vi "load_calib_file.vi"(0 "file_1":path, 1 "file_2":path, 2 "transpose? (F)":bool, 3 "delimiter (;)":string=";", 4 "format (%.3f)":string="%.3f") -> (5 "insieme":dbl[][](array[numeric]))   [LabVIEW 2021]
uses:
  <vilib>/Utility/file.llb/Read Delimited Spreadsheet (DBL).vi
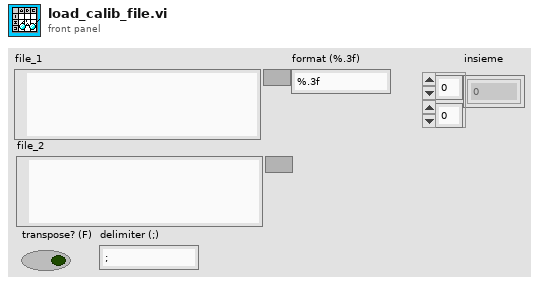
[diagram p1: front panel]
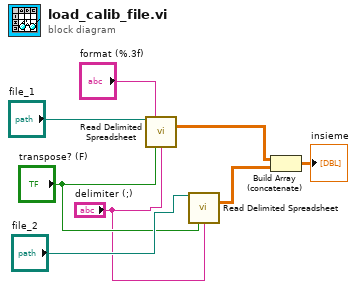
[diagram p0: block diagram]
diagram:
  n1 = call-poly <vilib>:"Read Delimited Spreadsheet.vi"("file path (dialog if empty)"="file_1", "format (%.3f)"="format (%.3f)", "transpose? (F)"="transpose? (F)", "delimiter (\\t)"="delimiter (;)") -> ("all rows"=w8:dbl[][])  [unwired: 6 in, 5 out]
  n2 = call-poly <vilib>:"Read Delimited Spreadsheet.vi"("file path (dialog if empty)"="file_2", "transpose? (F)"="transpose? (F)", "delimiter (\\t)"="delimiter (;)") -> ("all rows"=w7:dbl[][])  [unwired: 7 in, 5 out]
  n3 = Build Array (concatenate)(w8, w7) -> (→"insieme":dbl[][])
